vi "uTTA_LogSerial.vi"(6 "Data_Sent":string) -> ()   [LabVIEW 2021]
uses:
  uTTA_GV_Serial_Monitor.vi
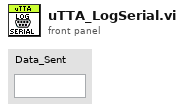
[diagram p1: front panel]
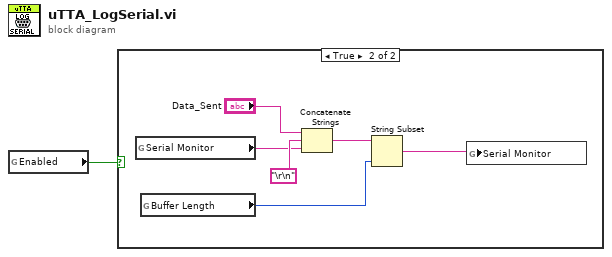
[diagram p0: block diagram]
diagram:
  n1 = global read "uTTA_GV_Serial_Monitor.vi" "Enabled"() -> (w1:bool)
  n2 = case shown="True" w1 {
    frame False {
    }
    frame True {
      n3 = global read "uTTA_GV_Serial_Monitor.vi" "Serial Monitor"() -> (w6:string)
      n4 = global read "uTTA_GV_Serial_Monitor.vi" "Buffer Length"() -> (w2:u32)
      n5 = Concatenate Strings("Data_Sent", "\r\n", w6) -> (w4:string)
      n6 = String Subset(string=w4, length (rest)=w2) -> (substring=w3:string)  [unwired: 1 in]
      n7 = global write "uTTA_GV_Serial_Monitor.vi" "Serial Monitor"(w3) -> ()
    }
  }
